vi "Config SMU-VSU selector.vi"(0 "VISA session":refnum<visa-resource-name>, 1 "I name (max 6 chars)":string, 2 "standby":bool, 3 "Range mode":u16(ring) items=["Auto", "Limited", "Fixed"], 5 "unit to configure":u32(slide) max=7 scale=0.0..7.0, 7 "function":u32(slide) max=4 scale=0.0..4.0, 9 "mode":u32(slide) max=4 scale=0.0..4.0, 11 "error in (no error)":errorcluster, 12 "V name (max 6 chars)":string, 13 "series resistance *":u32(slide) max=3 scale=0.0..3.0, 14 "Range":u8(slide)=6 max=11 scale=0.0..11.0) -> (4 "dup VISA resource name":refnum<visa-resource-name>, 6 "unit to configure (SMU)":u32(slide) max=5 scale=0.0..5.0, 8 "unit to configure (VSU)":u32(slide) max=5 scale=0.0..1.0, 15 "error out":errorcluster)   [LabVIEW 2016]
doc: "This VI is used to select the SMU or VSU to be configured."
panel:
  # "<--->"
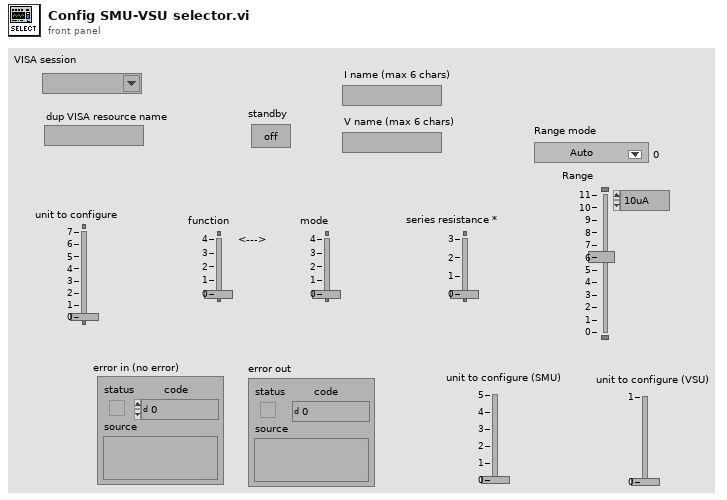
[diagram p1: front panel]
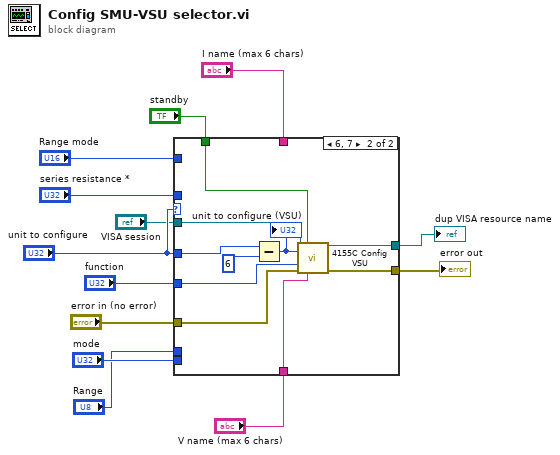
[diagram p0: block diagram]
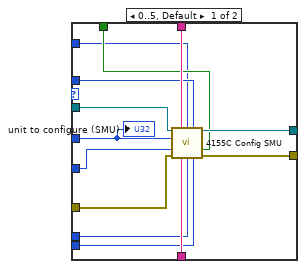
[diagram p2: hidden frame]
diagram:
  n1 = case shown="6, 7" "unit to configure" {
    tunnel: "unit to configure" -> [w14 w36]
    tunnel: "function" -> [w26 w33]
    tunnel: "error in (no error)" -> [w25 w29]
    tunnel: [w24 w31] -> w10
    tunnel: [w23 w32] -> w9
    tunnel: "I name (max 6 chars)" -> [w22 _]
    tunnel: "V name (max 6 chars)" -> [w21 w30]
    tunnel: "standby" -> [w20 w28]
    tunnel: "VISA session" -> [w19 w27]
    tunnel: "series resistance *" -> [w18 _]
    tunnel: "mode" -> [w17 _]
    tunnel: "Range mode" -> [w16 _]
    tunnel: "Range" -> [w15 _]
    frame 0..5, Default {
      n2 = call "4155C Config SMU.vi"("VISA session"=w19, "I name (max 6 chars)"=w22, "Range mode"=w16, "series resistance *"=w18, "unit to configure"=w14, "function"=w26, "standby"=w20, "error in (no error)"=w25, "V name (max 6 chars)"=w21, "Range"=w15, "mode"=w17) -> ("dup VISA resource name"=w23:refnum<visa-resource-name>, "error out"=w24:errorcluster)  [unwired: 3 in]
      "unit to configure (SMU)" <- w14
    }
    frame 6, 7 {
      n3 = Subtract(x=w36, y=u32 6) -> (x-y=w34:u32)
      "unit to configure (VSU)" <- w34
      n4 = call "4155C Config VSU.vi"("VISA session"=w27, "standby"=w28, "unit to configure"=w34, "function"=w33, "error in (no error)"=w29, "V name (max 6 chars)"=w30) -> ("dup VISA resource name"=w32:refnum<visa-resource-name>, "error out"=w31:errorcluster)  [unwired: 8 in]
    }
  }
  "dup VISA resource name" <- w9
  "error out" <- w10
